vi "Detect Target.vi"(0 "Image":T1, 1 "Image Mask":T1) -> (2 "Original Image":T1(plugin-control), 3 "X":i16, 4 "Y":i16, 5 "Found Target":bool)   [LabVIEW 2015]
uses:
  Camera Types.ctl
  <vilib>/vision/Image Controls.llb/IMAQ Image.ctl
  <vilib>/vision/NI_Vision_Development_Module.lvlib
panel:
  out "Highest Avg Score":dbl
  in  "Min Score Threshold":i32=75
  out "Detected Targets":T2(array[cluster]) {"Normalized Rect"."Numeric 5" format="%#_2g"; "Normalized Rect"."Numeric 3" format="%#_2g"; "Normalized Rect"."Numeric 2" format="%#_2g"; "Normalized Rect"."Numeric" format="%#_2g"}
  out "Sorted Particle Scores":T3(array[cluster]) {"Moment Factor" format="%#_3g"; "Aspect Ratio" format="%#_3g"; "Area to CH" format="%#_3g"; "X" format="%#_3g"; "Y" format="%#_3g"}
  in  "Display Mask":bool=TRUE
  in  "Emphasize Limit Tests":bool=TRUE
  in  "Camera Type":T4=enum."MS HD3000 square"
  in  "Aspect Fudge Factor":dbl=1.0
  out "Qualified Particles":i32
  in  "LED Color":T5={"Hue"={81.06675207900297, 16.56832035624079}, "Sat"={142.67857142857144, 255.0}, "Val"={103.21428571428572, 255.0}} {"Hue" scale=0.0..255.0 scale format="%#_3g"}
  out "Masked":T1(plugin-control)
  # "This is only the initial camera size.\nOther camera setup is done\non the diagram. Notice it is set\nonce before the loop but can be\nupdated within the loop if needed."
  # "Instructions:\nUse LED Color to threshold and build particles. Adjust calibration if needed.\nDisplays are very useful for debugging, but will slow down execution, so you\nmay want to disable once working.\nAnnotations show the rectangle and the scores from top to bottom.\nChange camera setting on diagram."
  # "Density Profile"
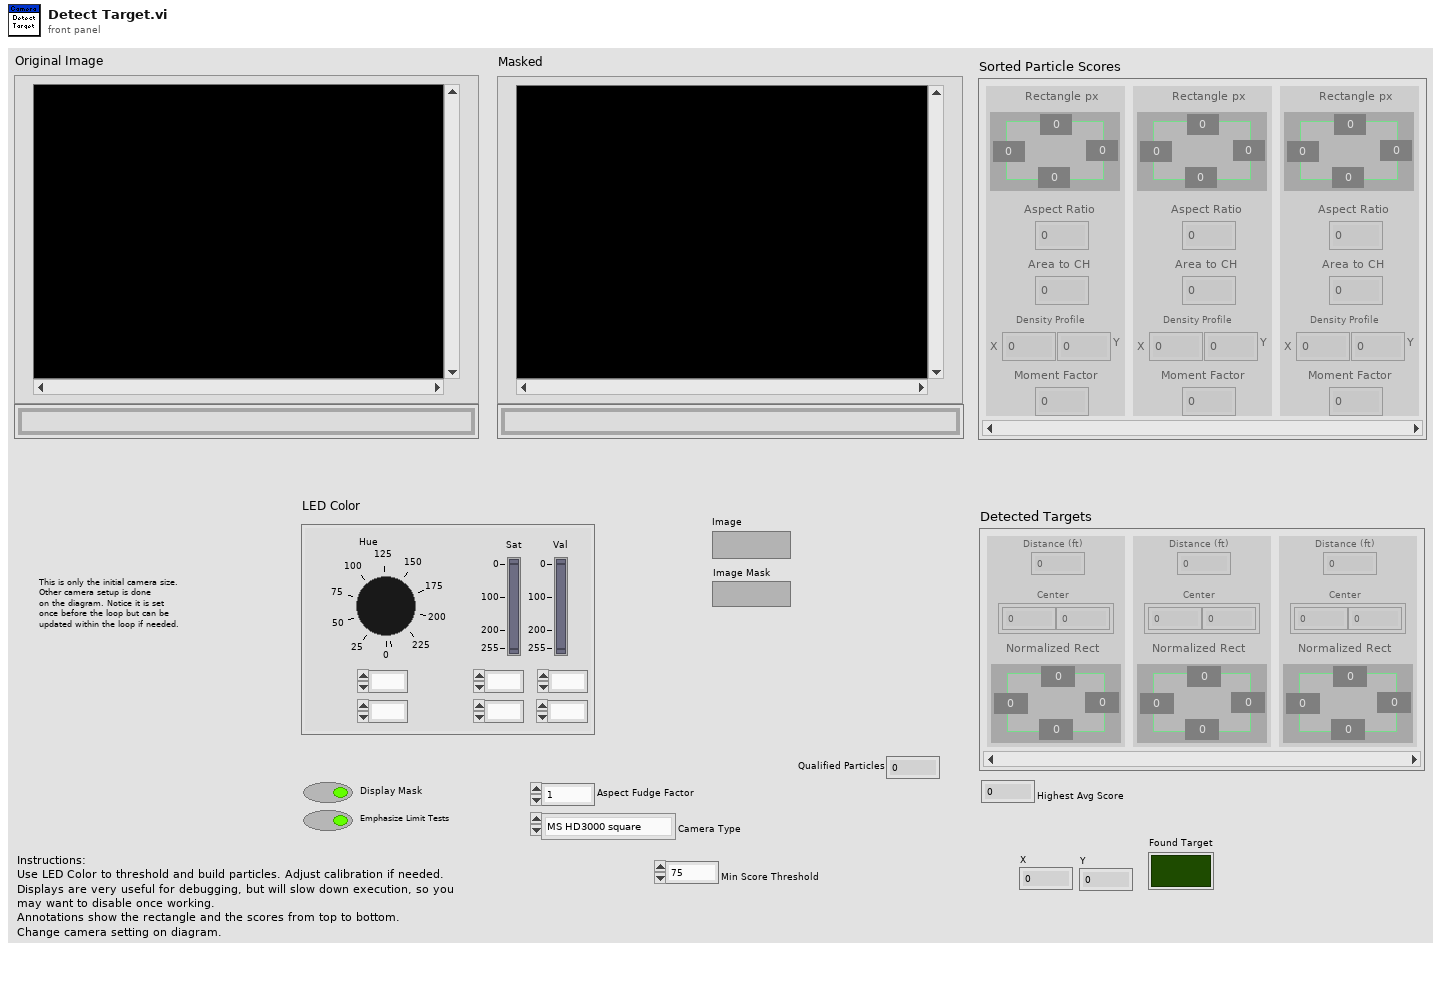
[diagram p1: front panel]
types:
  T1 = typedef "IMAQ Image.ctl" = refnum<image>
  T2 = cluster{"Distance (ft)":dbl, "Center":cluster{dbl, dbl}, "Normalized Rect":cluster{"Numeric":dbl, "Numeric 2":dbl, "Numeric 3":dbl, "Numeric 5":dbl}}[]
  T3 = cluster{"Rectangle px":cluster{"Numeric":dbl, "Numeric 2":dbl, "Numeric 3":dbl, "Numeric 5":dbl}, "Aspect Ratio":dbl, "Area to CH":dbl, "X":dbl, "Y":dbl, "Moment Factor":dbl}[]
  T4 = typedef "Camera Types.ctl" = enum16{"206", "1011", "1013", "MS HD3000 square", "MS HD3000 640x480"}
  T5 = cluster{"Hue":cluster{dbl, dbl}, "Sat":cluster{dbl, dbl}, "Val":cluster{dbl, dbl}}
  T6 = typedef "Particle Parameters" = i32
  T7 = cluster{"Bounding box":cluster{"left":dbl, "top":dbl, "right":dbl, "bottom":dbl}, "Aspect Ratio":dbl, "Area to CH":dbl, "X Mask":dbl, "Y Mask":dbl, "Moment":dbl}[]
  T8 = cluster{"Rectangle":cluster{"Numeric":dbl, "Numeric 2":dbl, "Numeric 3":dbl, "Numeric 5":dbl}, "L":dbl, "Area to CH":dbl, "X":dbl, "Y":dbl, "Moment Factor":dbl}[]
  T9 = cluster{"Rectangle":cluster{"Numeric":dbl, "Numeric 2":dbl, "Numeric 3":dbl, "Numeric 5":dbl}, "L":dbl, "Area to CH":dbl, "X":dbl, "Y":dbl, "Moment Factor":dbl}
  T10 = cluster{"Numeric":dbl, "Numeric 2":dbl, "Numeric 3":dbl, "Numeric 5":dbl}
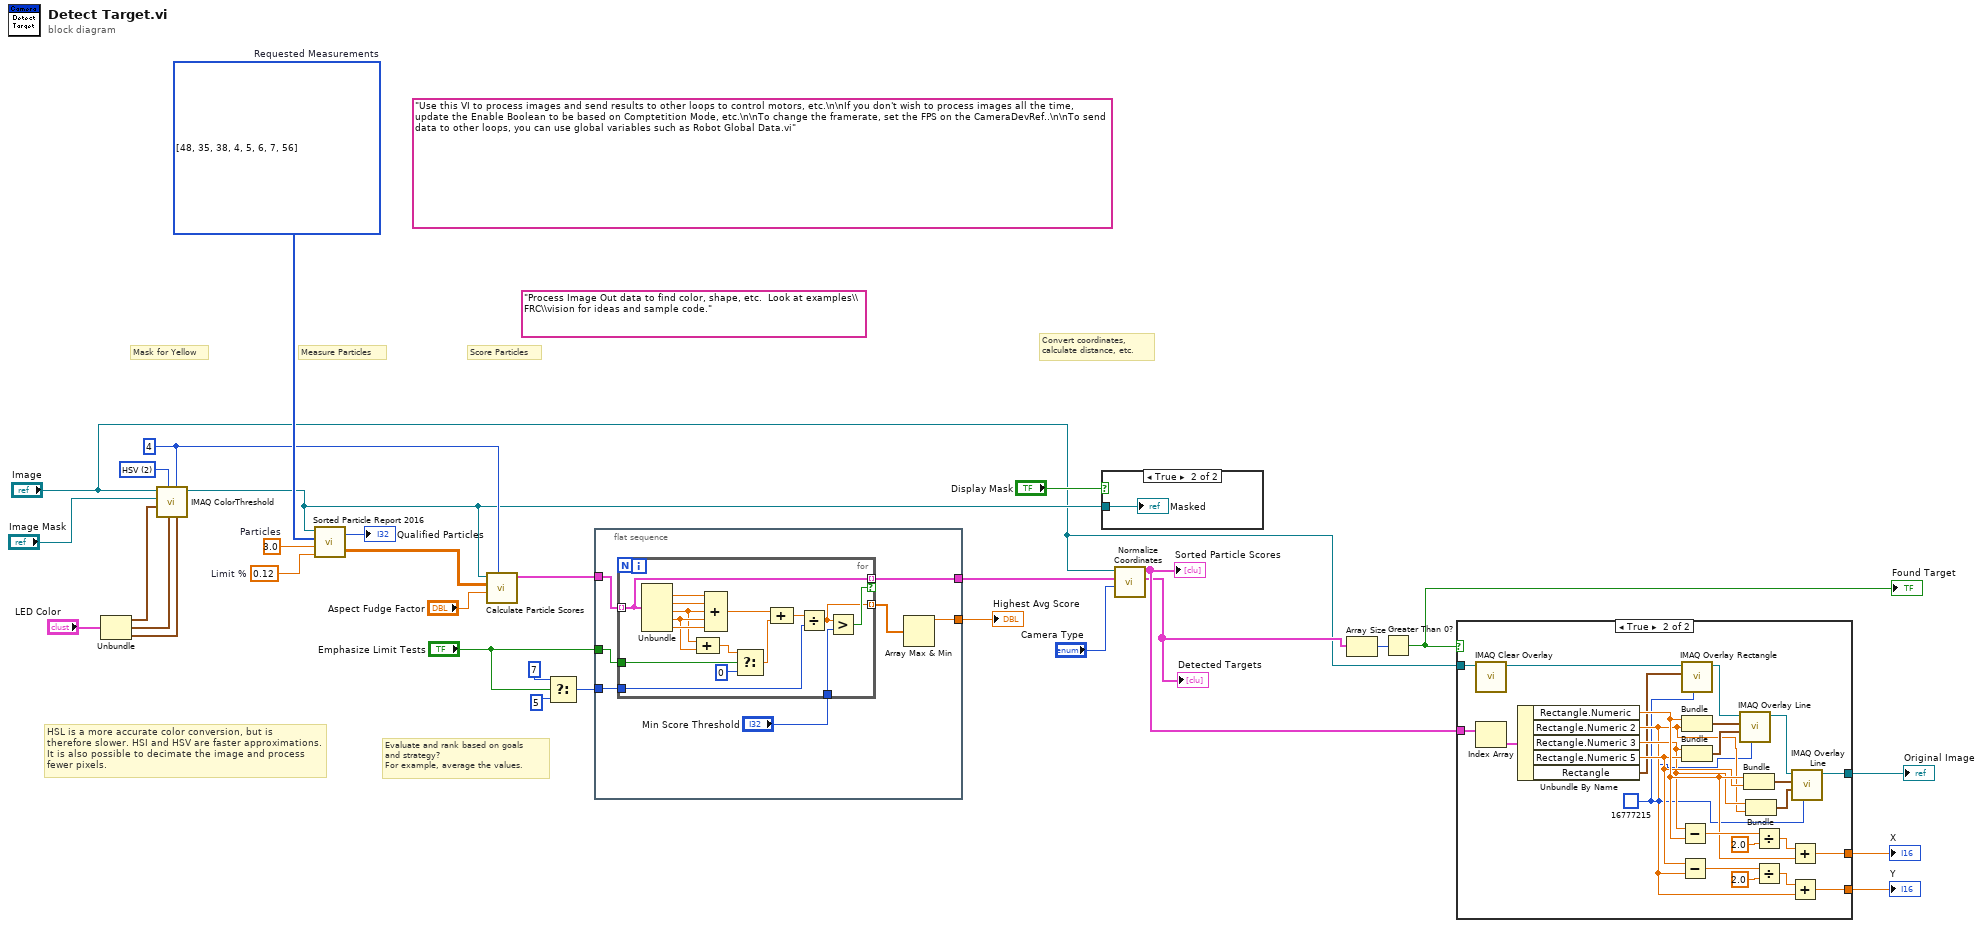
[diagram p0: block diagram]
diagram:
  w12 = 4 ("Replace Value")
  w22 = u16 2 items=["RGB", "HSL", "HSV", "HSI"] ("Color Mode")
  (unwired) "Process Image Out data to find color, shape, etc.  Look at examples\\FRC\\vision for ideas and sample code."
  w24 = 0.12  # Limit %
  w26 = 3.0  # Particles
  (unwired) "Use this VI to process images and send results to other loops to control motors, etc.\n\nIf you don't wish to process images all the time, update the Enable Boolean to be based on Comptetition Mode, etc.\n\nTo change the framerate, set the FPS on the CameraDevRef..\n\nTo send data to other loops, you can use global variables such as Robot Global Data.vi"
  w31 = T6[] [48, 35, 38, 4, 5, 6, 7, 56] items=["Center of Mass X", "Center of Mass Y", "First Pixel X", "First Pixel Y", "Bounding Rect Left", "Bounding Rect Top", "Bounding Rect Right", "Bounding Rect Bottom", "Max Feret Diameter Start X", "Max Feret Diameter Start Y", "Max Feret Diameter End X", "Max Feret Diameter End Y", "Max Horiz. Segment Length Left", "Max Horiz. Segment Length Right", "Max Horiz. Segment Length Row", "-", "Bounding Rect Width", "Bounding Rect Height", "Bounding Rect Diagonal", "Perimeter", "Convex Hull Perimeter", "Holes' Perimeter", "Max Feret Diameter", "Equivalent Ellipse Major Axis", "Equivalent Ellipse Minor Axis", "Equivalent Ellipse Minor Axis (Feret)", "Equivalent Rect Long Side", "Equivalent Rect Short Side", "Equivalent Rect Diagonal", "Equivalent Rect Short Side (Feret)", "Average Horiz. Segment Length", "Average Vert. Segment Length", "Hydraulic Radius", "Waddel Disk Diameter", "-", "Area", "Holes' Area", "Particle & Holes' Area", "Convex Hull Area", "Image Area", "-", "Number of Holes", "Number of Horiz. Segments", "Number of Vert. Segments", "-", "Orientation", "Max Feret Diameter Orientation", "-", "% Area/Image Area", "% Area/(Particle & Holes' Area)", "Ratio of Equivalent Ellipse Axes", "Ratio of Equivalent Rect Sides", "-", "Elongation Factor", "Compactness Factor", "Heywood Circularity Factor", "Type Factor", "-", "Sum X", "Sum Y", "Sum XX", "Sum XY", "Sum YY", "Sum XXX", "Sum XXY", "Sum XYY", "Sum YYY", "-", "Moment of Inertia XX", "Moment of Inertia XY", "Moment of Inertia YY", "Moment of Inertia XXX", "Moment of Inertia XXY", "Moment of Inertia XYY", "Moment of Inertia YYY", "Norm. Moment of Inertia XX", "Norm. Moment of Inertia XY", "Norm. Moment of Inertia YY", "Norm. Moment of Inertia XXX", "Norm. Moment of Inertia XXY", "Norm. Moment of Inertia XYY", "Norm. Moment of Inertia YYY", "Hu Moment 1", "Hu Moment 2", "Hu Moment 3", "Hu Moment 4", "Hu Moment 5", "Hu Moment 6", "Hu Moment 7"]  # Requested Measurements
  # "HSL is a more accurate color conversion, but is\ntherefore slower. HSI and HSV are faster approximations.\nIt is also possible to decimate the image and process\nfewer pixels."
  # "Evaluate and rank based on goals\nand strategy?\nFor example, average the values."
  # "Measure Particles"
  # "Convert coordinates,\ncalculate distance, etc."
  # "Score Particles"
  # "Mask for Yellow"
  n1 = Unbundle("LED Color") -> ("Hue"=w30:cluster{dbl, dbl}, "Sat"=w29:cluster{dbl, dbl}, "Val"=w28:cluster{dbl, dbl})
  n2 = call "IMAQ ColorThreshold"("Blue or Luma or Val or Inten Range"=w28, "Replace Value"=w12, "Green or Sat Range"=w29, "Color Mode"=w22, "Red or Hue Range"=w30, "Image Dst"="Image Mask", "Image Src"="Image") -> ("Image Dst Out"=w5:T1)  [unwired: 3 in, 1 out]
  n3 = call "Sorted Particle Report 2016.vi"("Min Area Size %"=w24, "Particle Count Limit"=w26, "Pixel Measurements"=w31, "Image in"=w5) -> ("Sorted Data"=w21:dbl[][], "Particles"=→"Qualified Particles":i32)
  n4 = call "Calculate Particle Scores.vi"("Pixel Value"=w12, "Aspect Fudge Factor"="Aspect Fudge Factor", "Sorted Data"=w21, "Image in"=w5) -> ("Scores"=w19:T7)  [unwired: 7 in]
  n5 = Select(t=7, s="Emphasize Limit Tests", f=5) -> (s? t:f=w16:i32)
  n6 = flat-sequence {
    tunnel: w19 -> [w37]
    tunnel: w16 -> [w35]
    tunnel: [w38] -> w15
    tunnel: [w32] -> w13
    tunnel: "Emphasize Limit Tests" -> [w36]
    frame #0 {
      n7 = for {
        tunnel: w37 -> [w52] mode=indexing
        tunnel: [w52] -> w32 mode=indexing if=w51
        tunnel: [w50] -> w33 mode=indexing
        tunnel: w35 -> [w49]
        tunnel: "Min Score Threshold" -> [w48]
        tunnel: w36 -> [w41]
        n8 = Unbundle(w52) -> ("Aspect Ratio"=w54:dbl, "Area to CH"=w53:dbl, "X Mask"=w43:dbl, "Y Mask"=w44:dbl, "Moment"=w45:dbl)  [unwired: 1 out]
        n9 = Compound Arithmetic op=ADD(w43, w44) -> (w42:dbl)
        n10 = Compound Arithmetic op=ADD(w54, w53, w43, w44, w45) -> (w47:dbl)
        n11 = Select(t=w42, s=w41, f=0) -> (s? t:f=w40:dbl)
        n12 = Compound Arithmetic op=ADD(w47, w40) -> (w46:dbl)
        n13 = Divide(x=w46, y=w49) -> (x/y=w50:dbl)
        n14 = Greater?(x=w50, y=w48) -> (0:w51:bool)
      }
      n15 = Array Max & Min(array=w33) -> (max value=w38:dbl)  [unwired: 3 out]
    }
  }
  n16 = case shown="True" "Display Mask" {
    tunnel: w5 -> [_ w55]
    frame False {
    }
    frame True {
      "Masked" <- w55
    }
  }
  n17 = call "Normalize Coordinates.vi"("Camera Type"="Camera Type", "Targets"=w13, "Image in"="Image") -> ("Found Targets"=w3:T2, "Sorted Scores"=w4:T8)  [unwired: 7 in]
  "Sorted Particle Scores" <- w4
  "Detected Targets" <- w3
  n18 = Array Size(array=w3) -> (size(s)=w9:i32)
  n19 = Greater Than 0?(x=w9) -> (x > 0?=w8:bool)
  "Found Target" <- w8
  n20 = case shown="True" w8 {
    tunnel: [_ w77] -> w7
    tunnel: [_ w73] -> w6
    tunnel: "Image" -> [w56 w71]
    tunnel: [w56 w66] -> w2
    tunnel: w4 -> [_ w58]
    frame False {
    }
    frame True {
      w59 = u32 16777215 ("Color")
      n21 = call "IMAQ Clear Overlay"("Image"=w71) -> ("Image Out"=w72:T1)  [unwired: 2 in, 8 out]
      n22 = Index Array(array=w58) -> (element=w81:T9)  [unwired: 1 in]
      n23 = Unbundle By Name(w81) -> ("Rectangle.Numeric"=w63:dbl, "Rectangle.Numeric 2"=w60:dbl, "Rectangle.Numeric 3"=w61:dbl, "Rectangle.Numeric 5"=w62:dbl, "Rectangle"=w57:T10)
      n24 = Subtract(x=w61, y=w63) -> (x-y=w79:dbl)
      n25 = Subtract(x=w62, y=w60) -> (x-y=w75:dbl)
      n26 = call "IMAQ Overlay Rectangle"("Color"=w59, "Rectangle"=w57, "Image"=w72) -> ("Image Out"=w70:T1)  [unwired: 7 in, 1 out]
      n27 = Bundle("Numeric"=w63, "Numeric 2"=w60) -> (w69:cluster{"Numeric":dbl, "Numeric 2":dbl})  [unwired: 1 in]
      n28 = Bundle("Numeric 3"=w61, "Numeric 5"=w62) -> (w68:cluster{"Numeric 3":dbl, "Numeric 5":dbl})  [unwired: 1 in]
      n29 = call "IMAQ Overlay Line"("Color"=w59, "End Point"=w68, "Start Point"=w69, "Image"=w70) -> ("Image Out"=w67:T1)  [unwired: 6 in, 1 out]
      n30 = Bundle("Numeric"=w63, "Numeric 5"=w62) -> (w65:cluster{"Numeric":dbl, "Numeric 5":dbl})  [unwired: 1 in]
      n31 = Bundle("Numeric 3"=w61, "Numeric 2"=w60) -> (w64:cluster{"Numeric 3":dbl, "Numeric 2":dbl})  [unwired: 1 in]
      n32 = Divide(x=w79, y=2.0) -> (x/y=w78:dbl)
      n33 = Divide(x=w75, y=2.0) -> (x/y=w74:dbl)
      n34 = Add(x=w78, y=w63) -> (x+y=w77:dbl)
      n35 = Add(x=w74, y=w60) -> (x+y=w73:dbl)
      n36 = call "IMAQ Overlay Line"("Color"=w59, "End Point"=w64, "Start Point"=w65, "Image"=w67) -> ("Image Out"=w66:T1)  [unwired: 6 in, 1 out]
    }
  }
  "X" <- w7
  "Y" <- w6
  "Original Image" <- w2
  "Highest Avg Score" <- w15
